vi "ATSh_Busy.vi"(11 "Handle":u32) -> (0 "Return Code":u32, 2 "Busy":bool, 3 "Handle_Out":u32)   [LabVIEW 2015]
doc: "_____AlazarTech, Scope_____\n\nQuery the devices's busy status.\nHandle input."
uses:
  ATSApi.dll
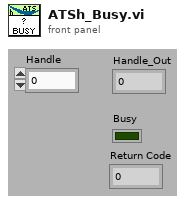
[diagram p1: front panel]
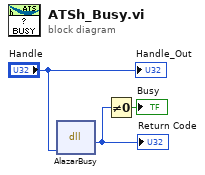
[diagram p0: block diagram]
diagram:
  n1 = dll-call lib="C:/IntensityOCT/trunk/ATSApi.dll" fn="AlazarBusy"("h"="Handle") -> (w3:u32)  [unwired: 4 in, 2 out]
  "Return Code" <- w3
  n2 = Not Equal To 0?(x=w3) -> (x != 0?=→"Busy":bool)
  "Handle_Out" <- "Handle"
